vi "BasicReadoutV775_noQDC.vi"() -> ()   [LabVIEW 2014]
uses:
  Program Files (x86)/CAEN/Comm/labview/CAENComm.lvlib
panel:
  out "Loop Counter":i32
  out "Event Counter":u32
  out "# Data":i32
  out "TDC Raw":u32[](array[numeric]) format="%.0b"
  out "Results":T1(array[cluster]) {"GeoAddr" format="%.0x"}
  in  "stop":bool
  out "TDC Histogram":u16[](graph)
  out "error out":errorcluster
  in  "Channel for hist":u8=30
  out "Decode time":dbl
  in  "Low Range threshold":u16
  in  "VME Base Address":u32=4026597376 format="%.0x"
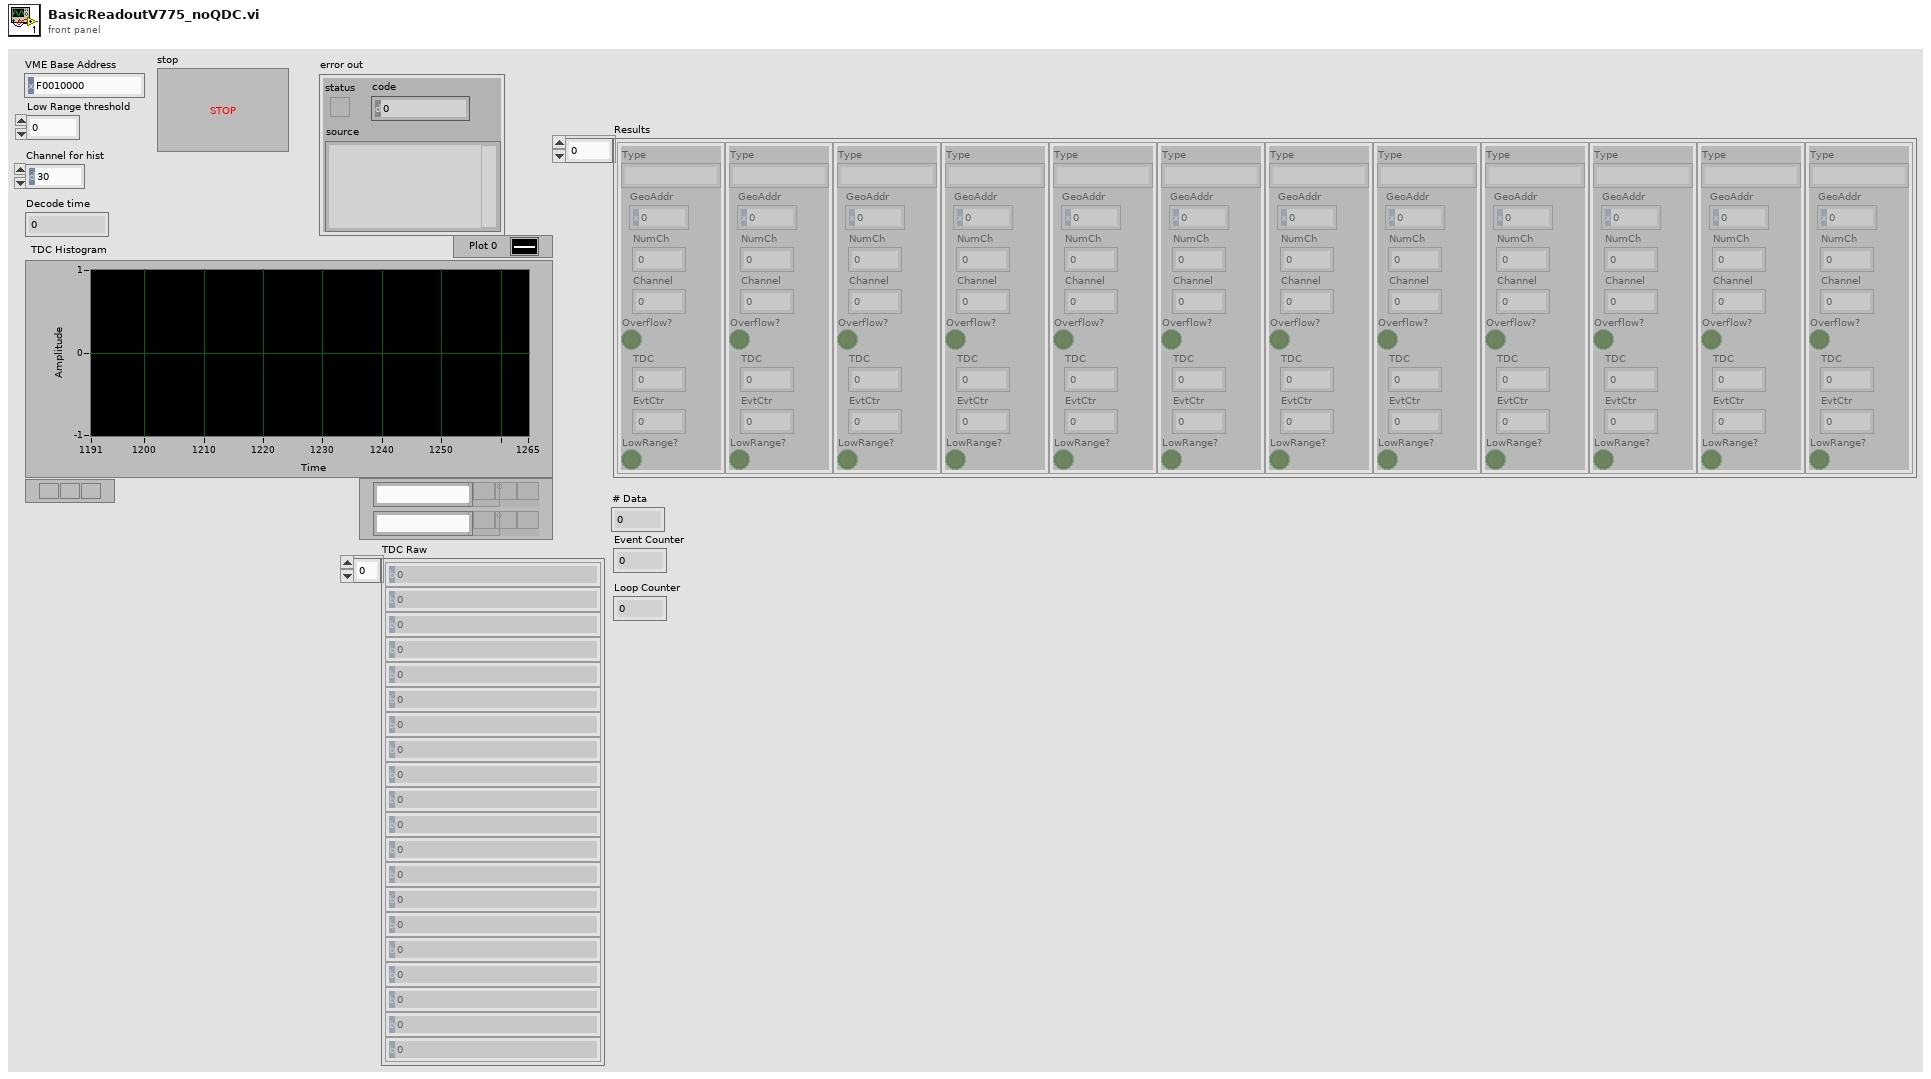
[diagram p1: front panel]
types:
  T1 = cluster{"Type":string, "GeoAddr":u8, "NumCh":u8, "Channel":u8, "Overflow?":bool, "TDC":u16, "EvtCtr":u32, "LowRange?":bool}[]
  T2 = cluster{"Type":string, "GeoAddr":u8, "NumCh":u8, "Channel":u8, "Overflow?":bool, "QDC":u16, "EvtCtr":u32, "Underflow?":bool}[]
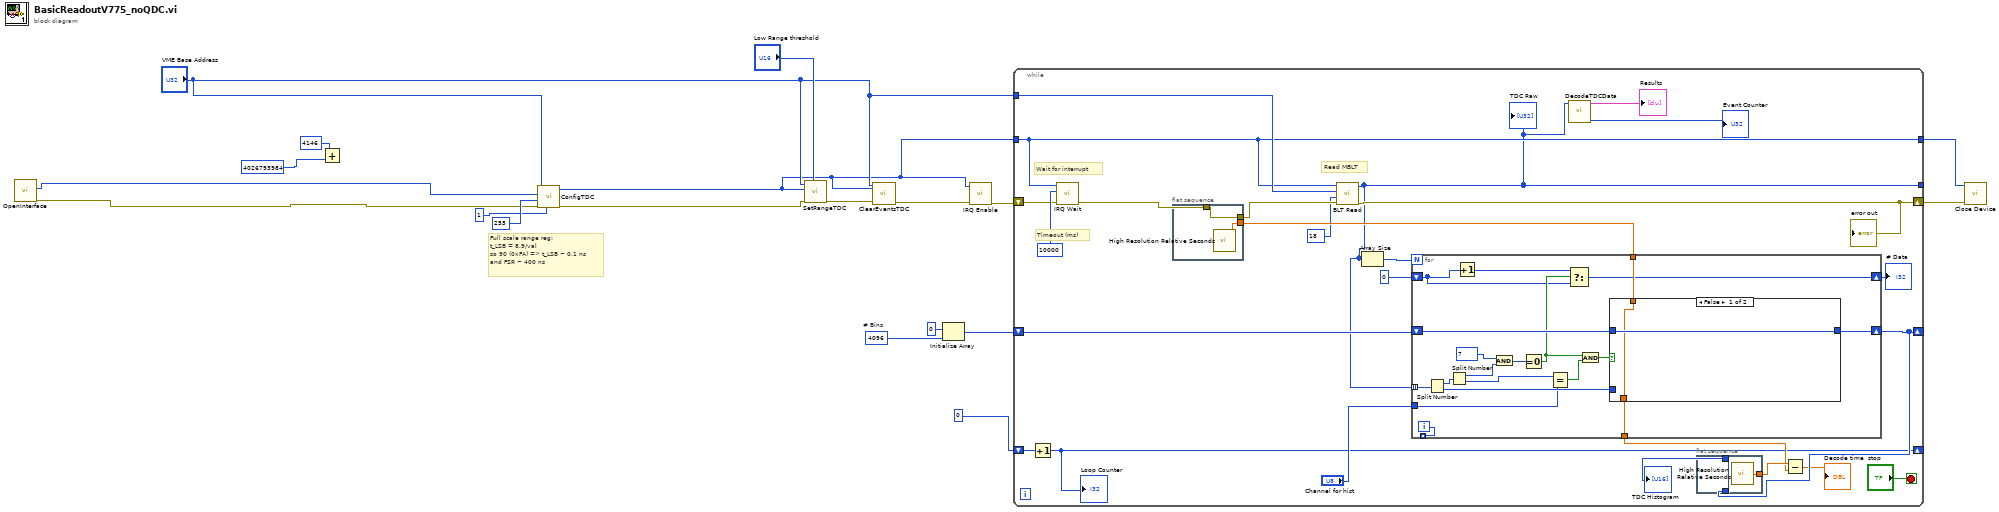
[diagram p0: block diagram]
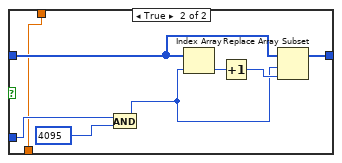
[diagram p2: hidden frame]
diagram:
  w14 = u16 4096  # # Bins
  # "Full scale range reg:\nt_LSB = 8.9/val\nso 90 (0xFA) => t_LSB ~ 0.1 ns\nand FSR ~ 400 ns"
  n1 = call "OpenInterface.vi"() -> ("error out"=w3:errorcluster, "handle"=w8:i32)  [unwired: 9 in, 1 out]
  n2 = Add(x=u32 4146, y=u32 4026793984 ("VME module Base Address")) -> ()  [unwired: 1 out]
  n3 = call "ConfigTDC.vi"("# Evts to Acquire"=u16 1 ("# of events before transfer (max 32)"), "error in (no error)"=w3, "FSR setting"=u16 255 ("Data"), "handle"=w8, "VME Base Address"="VME Base Address") -> ("error out"=w19:errorcluster, "handle out"=w1:i32)  [unwired: 5 in]
  n4 = call "SetRangeTDC.vi"("Low Range threshold"="Low Range threshold", "error in (no error)"=w19, "handle"=w1, "VME module Base Address"="VME Base Address") -> ("error out"=w17:errorcluster)  [unwired: 7 in]
  n5 = call "ClearEventsTDC.vi"("error in (no error)"=w17, "handle"=w1, "VME module Base Address"="VME Base Address") -> ("error out"=w2:errorcluster)  [unwired: 6 in, 2 out]
  n6 = Initialize Array(u16 0 ("element"), w14) -> (w16:u16[])
  n7 = call "IRQ Enable.vi"("error in (no error)"=w2, "handle"=w1) -> ("error out"=w13:errorcluster)  [unwired: 9 in]
  n8 = while {
    tunnel: "VME Base Address" -> [w23]
    tunnel: [w21] -> _
    shift-right: [w25] -> w11
    shift-left: w13 -> [w33]
    shift-right: [w40] -> _
    shift-left: w16 -> [w44]
    tunnel: w1 -> [w22]
    tunnel: [w22] -> w10
    shift-right: [w27] -> _
    shift-left: 0 -> [w28]
    stop <- "stop" stop-if-true
    # "Read MBLT"
    # "Wait for interrupt"
    # "Timeout (ms)"
    n9 = Increment(x=w28) -> (x+1=w27:i32)
    "Loop Counter" <- w27
    n10 = call "IRQ Wait.vi"("error in (no error)"=w33, "Timeout"=u32 10000, "handle"=w22) -> ("error out"=w20:errorcluster)  [unwired: 8 in]
    n11 = flat-sequence {
      tunnel: [w46] -> w26
      tunnel: w20 -> [w46]
      tunnel: [w45] -> w34
      frame #0 {
        n12 = call <vilib>:"High Resolution Relative Seconds.vi"() -> ("relative seconds"=w45:dbl)
      }
    }
    n13 = call "BLT Read.vi"("error in (no error)"=w26, "BltSize"=18, "Address"=w23, "handle"=w22) -> ("error out"=w25:errorcluster, "Buff"=w21:u32[])  [unwired: 5 in, 1 out]
    "error out" <- w25
    "TDC Raw" <- w21
    n14 = Array Size(array=w21) -> (size(s)=w35:i32)
    n15 = for {
      N: w35 -> [_]
      tunnel: w21 -> [w65] mode=indexing
      shift-right: [w56] -> w40
      shift-left: w44 -> [w57]
      tunnel: "Channel for hist" -> [w55]
      tunnel: w34 -> [w54]
      tunnel: [w53] -> w37
      shift-right: [w48] -> w30
      shift-left: 0 -> [w50]
      tunnel: [w47] -> _ mode=indexing
      i -> [w47]
      n16 = Split Number(x=w65) -> (hi(x)=w64:u16, lo(x)=w61:u16)
      n17 = Split Number(x=w64) -> (hi(x)=w60:u8, lo(x)=w52:u8)
      n18 = Increment(x=w50) -> (x+1=w49:i32)
      n19 = And(x=u8 7, y=w60) -> (x .and. y?=w62:u8)
      n20 = Equal To 0?(x=w62) -> (x = 0?=w51:bool)
      n21 = Equal?(x=w52, y=w55) -> (x = y?=w58:bool)
      n22 = Select(t=w49, s=w51, f=w50) -> (s? t:f=w48:i32)
      n23 = And(x=w51, y=w58) -> (x .and. y?=w59:bool)
      n24 = case shown="False" w59 {
        tunnel: w61 -> [_ w74]
        tunnel: w57 -> [w67 w72]
        tunnel: [w67 w70] -> w56
        tunnel: w54 -> [w66 w69]
        tunnel: [w66 w69] -> w53
        frame False {
        }
        frame True {
          n25 = And(x=w74, y=u16 4095) -> (x .and. y?=w68:u16)
          n26 = Index Array(array=w72, index=w68) -> (element=w73:u16)
          n27 = Increment(x=w73) -> (x+1=w71:u16)
          n28 = Replace Array Subset(array=w72, new element=w71, index=w68) -> (w70:u16[])
        }
      }
    }
    "# Data" <- w30
    n29 = call "DecodeTDCData.vi"("Buff"=w21) -> ("Event Counter"=→"Event Counter":u32, "Array"=→"Results":T2)  [unwired: 8 in, 1 out]
    n30 = flat-sequence {
      tunnel: w40 -> [w77]
      tunnel: [w77] -> w39
      tunnel: [w76] -> w38
      frame #0 {
        n31 = call <vilib>:"High Resolution Relative Seconds.vi"() -> ("relative seconds"=w76:dbl)
      }
    }
    n32 = Subtract(x=w38, y=w37) -> (x-y=→"Decode time":dbl)
    "TDC Histogram" <- w39
  }
  n33 = call "Close Device.vi"("error in (no error)"=w11, "handle"=w10) -> ()  [unwired: 9 in, 1 out]
